vi "Set Combobox Items.vi"(6 "Combo Box Ref":refnum<vi>, 8 "error in (no error)":errorcluster, 9 "Run Mode?":bool, 10 "Indicator?":bool, 11 "Path Selector in":refnum<class "MGI Path Selector.lvclass">) -> (0 "error out":errorcluster, 2 "Strings And Values []":T1, 3 "Path Selector out":refnum<class "MGI Path Selector.lvclass">)   [LabVIEW 2020, in "MGI Path Selector.lvclass"]
doc: "Sets the Combobox strings to appropriate values for the specified state of the XControl.\n\nAuthored by Shawn Walpole\nsupport@mooregoodideas.com\nwww.mooregoodideas.com\n\nCopyright (c) 2013, Moore Good Ideas, Inc.\n\nAll rights reserved.\n\nRedistribution and use in source and binary forms, with or without modification, are permitted provided that the following conditions are met:\n\n * Redistributions of source code must retain the above copyright notice, this list of conditions and the following disclaimer.\n * Redistributions in binary form must reproduce the above copyright notice, this list of conditions and the following disclaimer in the documentation and/or other materials provided with the distribution.\n * Neither the name of Moore Good Ideas, Inc. nor the names of its contributors may be used to endorse or promote products derived from this software without specific prior written permission.\n\nTHIS SOFTWARE IS PROVIDED BY THE COPYRIGHT HOLDERS AND CONTRIBUTORS \"AS IS\" AND ANY EXPRESS OR IMPLIED WARRANTIES, INCLUDING, BUT NOT LIMITED TO, THE IMPLIED WARRANTIES OF MERCHANTABILITY AND FITNESS FOR A PARTICULAR PURPOSE ARE DISCLAIMED. IN NO EVENT SHALL THE COPYRIGHT OWNER OR CONTRIBUTORS BE LIABLE FOR ANY DIRECT, INDIRECT, INCIDENTAL, SPECIAL, EXEMPLARY, OR CONSEQUENTIAL DAMAGES (INCLUDING, BUT NOT LIMITED TO, PROCUREMENT OF SUBSTITUTE GOODS OR SERVICES; LOSS OF USE, DATA, OR PROFITS; OR BUSINESS INTERRUPTION) HOWEVER CAUSED AND ON ANY THEORY OF LIABILITY, WHETHER IN CONTRACT, STRICT LIABILITY, OR TORT (INCLUDING NEGLIGENCE OR OTHERWISE) ARISING IN ANY WAY OUT OF THE USE OF THIS SOFTWARE, EVEN IF ADVISED OF THE POSSIBILITY OF SUCH DAMAGE."
uses:
  <userlib>/_MGI/User Interface/Path Selector XControl/Class Hierarchy/MGI Path Selector.lvclass
  <vilib>/Utility/miscctls.llb/LVComboBoxStrsAndValuesArrayTypeDef.ctl
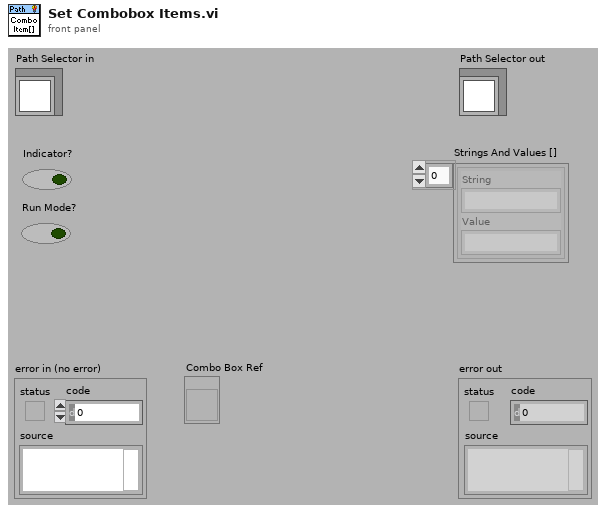
[diagram p1: front panel]
types:
  T1 = typedef "LVComboBoxStrsAndValuesArrayTypeDef.ctl" = cluster{"String":string, "Value":string}[]
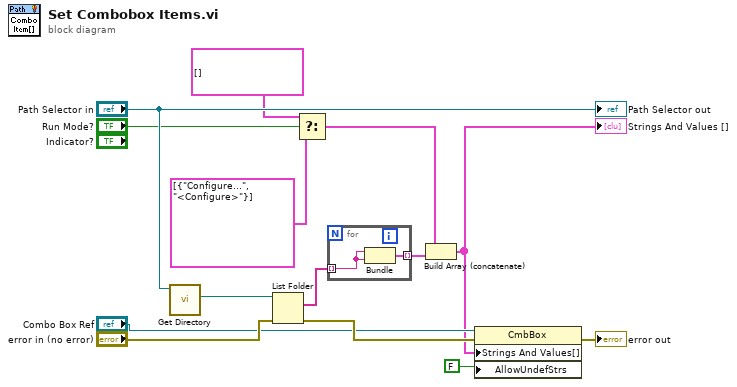
[diagram p0: block diagram]
diagram:
  n1 = call-dynamic "Get Directory.vi"("Path Selector in"="Path Selector in") -> ("Start Path"=w7:path)  [unwired: 9 in, 1 out]
  n2 = List Folder(path=w7, error in="error in (no error)") -> (filenames=w1:string[], error out=w11:errorcluster)  [unwired: 2 in, 2 out]
  n3 = Select(t=cluster{string, string}[] [] ("element"), s="Run Mode?", f=cluster{string, string}[] [{"Configure...", "<Configure>"}] ("element")) -> (s? t:f=w4:cluster{string, string}[])
  n4 = for {
    tunnel: [w16] -> w8 mode=indexing
    tunnel: w1 -> [w15] mode=indexing
    n5 = Bundle(w15, w15) -> (w16:cluster{string, string})  [unwired: 1 in]
  }
  n6 = Build Array (concatenate)(w4, w8) -> (w9:cluster{string, string}[])
  "Strings And Values []" <- w9
  n7 = property class="CmbBox"(reference="Combo Box Ref", error in=w11, "Strings And Values[]"=w9, "AllowUndefStrs"=FALSE ("Allow Undefined Strings")) -> (error out=→"error out":errorcluster)  [unwired: 1 out]
  "Path Selector out" <- "Path Selector in"
